vi "wait_&_ackComando.vi"(8 "error in (no error)":errorcluster, 10 "?":T1=enum."FH", 11 "VISA Refnum in":refnum<visa-resource-name>) -> (0 "error out":errorcluster, 1 "Movimiento realizado?":bool)   [LabVIEW 2019, in "SHARED VI'S.lvlib"]
uses:
  SHARED VI'S.lvlib
  LVPROJ_MOVIMIENTO_CABEZAL/LABVIEW_MOVIMIENTO/MOVIMIENTO CABEZAL/Typedefs/Comandos.ctl
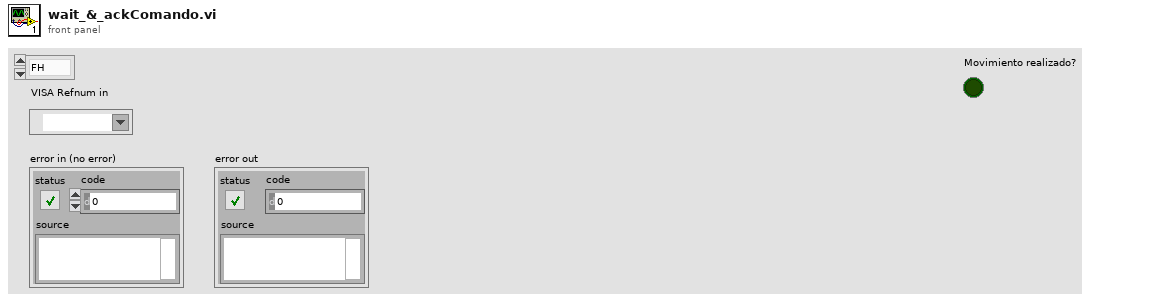
[diagram p1: front panel]
types:
  T1 = typedef "Comandos.ctl" = enum16{"H", "FH", "FM", "FI", "FX", "FY", "FZ", "I", "OK"}
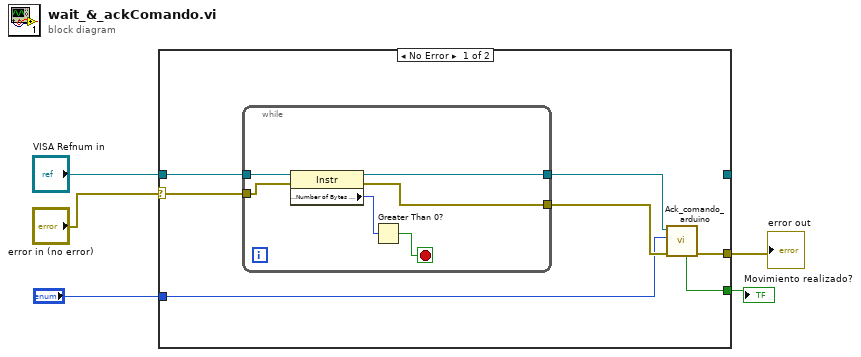
[diagram p0: block diagram]
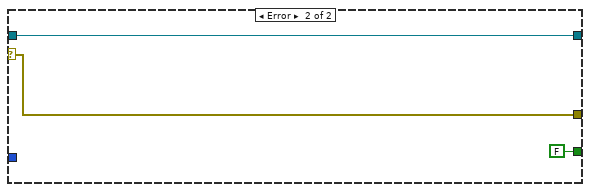
[diagram p2: hidden frame]
diagram:
  n1 = case shown="No Error" "error in (no error)" {
    selector: "error in (no error)" -> [w7 w21]
    tunnel: [w12 w21] -> w5
    tunnel: "VISA Refnum in" -> [w11 w20]
    tunnel: "?" -> [w8 _]
    tunnel: [_ w20] -> _
    tunnel: [w6 FALSE ("Movimiento realizado?")] -> w1
    frame No Error {
      n2 = while {
        tunnel: [w18] -> w9
        tunnel: w11 -> [w16]
        tunnel: [w15] -> w10
        tunnel: w7 -> [w13]
        stop <- w17 stop-if-true
        n3 = property class="Instr"(reference=w16, error in=w13) -> (reference out=w15:refnum<visa-resource-name>, error out=w18:errorcluster, "Serial Settings:Number of Bytes at Serial Port"=w14:u32)
        n4 = Greater Than 0?(x=w14) -> (x > 0?=w17:bool)
      }
      n5 = call "Ack_comando_arduino.vi"("error in (no error)"=w9, 10:w8, "VISA resource name"=w10) -> ("error IO"=w12:errorcluster, "Movimiento realizado?"=w6:bool)  [unwired: 6 in, 1 out]
    }
    frame Error {
    }
  }
  "error out" <- w5
  "Movimiento realizado?" <- w1
